vi "Main.vi"(7 "sweep rate, /min":dbl=0.2, 8 "sweep to:":dbl=-0.5, 9 "sweep":T6(radio)=enum."time_sweep") -> ()   [LabVIEW 2017] (continued)
                  n4093 = property on="data" class="Arr (strict)"() -> ("Value"=w5493:dbl[])  [unwired: 2 in, 2 out]
                  n4094 = case shown="True" w5491 {
                    tunnel: w5493 -> [w5494 w5497]
                    tunnel: [w5494 w5496] -> w5492
                    frame False {
                      # "We are not recording Step Value if it is linetrace"
                    }
                    frame True {
                      # "We are recording Step Value if it is mapping"
                      n4095 = property on="Current Hyper Value" class="DigNum (strict)"() -> ("Value"=w5495:dbl)  [unwired: 2 in, 2 out]
                      n4096 = Build Array (concatenate)(w5497, w5495) -> (w5496:dbl[])
                    }
                  }
                  n4097 = property on="data" class="Arr (strict)"("Value"=w5492) -> ()  [unwired: 2 in, 2 out]
                }
                frame #51 {
                  # "Record Step Value \nif it is mapping"
                  n4098 = property on="SuperHyper" class="Bool (strict)"() -> ("Value"=w5498:bool)  [unwired: 2 in, 2 out]
                  n4099 = property on="data" class="Arr (strict)"() -> ("Value"=w5500:dbl[])  [unwired: 2 in, 2 out]
                  n4100 = case shown="True" w5498 {
                    tunnel: w5500 -> [w5501 w5504]
                    tunnel: [w5501 w5503] -> w5499
                    frame False {
                      # "We are not recording Step Value if it is linetrace"
                    }
                    frame True {
                      # "We are recording SuperHyper_step if it is mapping"
                      n4101 = property on="Current SuperHyper Value" class="DigNum (strict)"() -> ("Value"=w5502:dbl)  [unwired: 2 in, 2 out]
                      n4102 = Build Array (concatenate)(w5504, w5502) -> (w5503:dbl[])
                    }
                  }
                  n4103 = property on="data" class="Arr (strict)"("Value"=w5499) -> ()  [unwired: 2 in, 2 out]
                }
              }
            }
            frame #4 {
              n4104 = property on="data" class="Arr (strict)"() -> ("Value"=w5505:dbl[])  [unwired: 2 in, 2 out]
            }
          }
          n4105 = stacked-sequence "add data to array" {
            tunnel: w4728 -> [w4740]
            tunnel: [w4739] -> w4727
            tunnel: w4726 -> [w4738]
            frame #0 {
              n4106 = Build Array (concatenate)(w4740, w4738) -> (w4739:dbl[][])
            }
          }
          n4107 = stacked-sequence "plot selected measurements" {
            seq-local: [_ w4763 _] -> [_ _ w4808]
            seq-local: [_ w4762 _] -> [_ _ w4809]
            tunnel: w4727 -> [_ w4761 _]
            frame #0 {
              n4108 = property on="XY Graph" class="XYGraph (strict)"("ActYScl"=0 ("Active Y Scale")) -> (error out=w4746:errorcluster)  [unwired: 2 in, 1 out]
              n4109 = property on="Show cursor" class="Bool (strict)"() -> ("Value"=w4741:bool)  [unwired: 2 in, 2 out]
              n4110 = property on="Xaxis" class="Ring (strict)"() -> ("Value"=w4751:u16)  [unwired: 2 in, 2 out]
              n4111 = property on="Yaxis" class="Ring (strict)"(error in=w4746) -> (error out=w4745:errorcluster, "RingText.Text"=w4744:string)  [unwired: 1 in, 1 out]
              n4112 = property on="XY Graph" class="XYGraph (strict)"("Cursor.Visible"=w4741) -> ()  [unwired: 2 in, 2 out]
              n4113 = property on="Figure_axis" class="Arr (strict)"() -> ("Value"=w4752:string[])  [unwired: 2 in, 2 out]
              n4114 = property on="XY Graph" class="XYGraph (strict)"(error in=w4745, "YScale.NameLbl.Text"=w4744) -> (error out=w4742:errorcluster)  [unwired: 1 in, 1 out]
              n4115 = property on="XY Graph" class="XYGraph (strict)"(error in=w4742, "ActYScl"=1 ("Active Y Scale")) -> (error out=w4748:errorcluster)  [unwired: 1 in, 1 out]
              n4116 = property on="Yright" class="Ring (strict)"(error in=w4748) -> (error out=w4749:errorcluster, "RingText.Text"=w4743:string)  [unwired: 1 in, 1 out]
              n4117 = Index Array(array=w4752, index=w4751) -> (element=w4753:string)
              n4118 = property on="XY Graph" class="XYGraph (strict)"("XScale.NameLbl.Text"=w4753) -> ()  [unwired: 2 in, 2 out]
              n4119 = property on="XY Graph" class="XYGraph (strict)"(error in=w4749, "YScale.NameLbl.Text"=w4743) -> ()  [unwired: 1 in, 2 out]
            }
            frame #1 {
              n4120 = local read "Xaxis"() -> (w4766:u16)
              n4121 = property on="Yright" class="Ring (strict)"() -> ("Value"=w4760:u16)  [unwired: 2 in, 2 out]
              n4122 = property on="Yright" class="Ring (strict)"() -> ("RingText.Text"=w4759:string)  [unwired: 2 in, 2 out]
              n4123 = property on="Xaxis" class="Ring (strict)"() -> ("RingText.Text"=w4765:string)  [unwired: 2 in, 2 out]
              n4124 = property on="Yaxis" class="Ring (strict)"() -> ("RingText.Text"=w4764:string)  [unwired: 2 in, 2 out]
              n4125 = local read "Yaxis"() -> (w4767:u16)
              n4126 = case shown="\"formula\"" w4759 {
                tunnel: [w4772 w4779] -> w4757
                tunnel: w4760 -> [_ w4778]
                tunnel: w4761 -> [w4773 w4777]
                tunnel: [w4771 errorcluster {"status"=FALSE, "code"=0, "source"=""} ("error out")] -> _
                frame "formula" {
                  n4127 = local read "formula_variables"() -> (w4774:string[])
                  n4128 = Transpose 2D Array(2D array=w4773) -> (transposed array=w4775:dbl[][])
                  n4129 = property on="Y_right_formula" class="Str"() -> ("Value"=w4770:string)  [unwired: 2 in, 2 out]
                  n4130 = call <vilib>:"Eval Multi-Variable Array.vi"("Variables"=w4774, "X Values"=w4775, "formula"=w4770) -> ("error out"=w4771:errorcluster, "Y Values"=w4772:dbl[])  [unwired: 1 in]
                }
                frame "0", Default {
                  n4131 = Index Array(array=w4777, index (col)=w4778) -> (element=w4779:dbl[])  [unwired: 1 in]
                }
              }
              n4132 = case shown="\"formula\"" w4765 {
                tunnel: [w4790 w4795] -> w4769
                tunnel: w4766 -> [w4793 _]
                tunnel: w4761 -> [w4792 w4799]
                tunnel: [errorcluster {"status"=FALSE, "code"=0, "source"=""} ("error out") w4796] -> w4763
                tunnel: [w4790 w4795] -> w4758
                frame "0", Default {
                  n4133 = Index Array(array=w4792, index (col)=w4793) -> (element=w4790:dbl[])  [unwired: 1 in]
                }
                frame "formula" {
                  n4134 = local read "formula_variables"() -> (w4798:string[])
                  n4135 = Transpose 2D Array(2D array=w4799) -> (transposed array=w4797:dbl[][])
                  n4136 = property on="X_axis_formula" class="Str"() -> ("Value"=w4794:string)  [unwired: 2 in, 2 out]
                  n4137 = call <vilib>:"Eval Multi-Variable Array.vi"("Variables"=w4798, "X Values"=w4797, "formula"=w4794) -> ("error out"=w4796:errorcluster, "Y Values"=w4795:dbl[])  [unwired: 1 in]
                }
              }
              n4138 = case shown="\"formula\"" w4764 {
                tunnel: [w4782 w4789] -> w4768
                tunnel: w4767 -> [_ w4788]
                tunnel: w4761 -> [w4783 w4787]
                tunnel: [w4781 errorcluster {"status"=FALSE, "code"=0, "source"=""} ("error out")] -> w4762
                frame "formula" {
                  n4139 = local read "formula_variables"() -> (w4784:string[])
                  n4140 = Transpose 2D Array(2D array=w4783) -> (transposed array=w4785:dbl[][])
                  n4141 = property on="Y_left_formula" class="Str"() -> ("Value"=w4780:string)  [unwired: 2 in, 2 out]
                  n4142 = call <vilib>:"Eval Multi-Variable Array.vi"("Variables"=w4784, "X Values"=w4785, "formula"=w4780) -> ("error out"=w4781:errorcluster, "Y Values"=w4782:dbl[])  [unwired: 1 in]
                }
                frame "0", Default {
                  n4143 = Index Array(array=w4787, index (col)=w4788) -> (element=w4789:dbl[])  [unwired: 1 in]
                }
              }
              n4144 = Bundle("Y Values"=w4769, "Y Values"=w4768) -> (w4756:cluster{"Y Values":dbl[], "Y Values":dbl[]})  [unwired: 1 in]
              n4145 = Bundle("Y Values"=w4758, "Y Values"=w4757) -> (w4755:cluster{"Y Values":dbl[], "Y Values":dbl[]})  [unwired: 1 in]
              n4146 = Build Array(w4756, w4755) -> (w4754:cluster{"Y Values":dbl[], "Y Values":dbl[]}[])
              n4147 = property on="XY Graph" class="XYGraph (strict)"("Value"=w4754) -> ()  [unwired: 2 in, 2 out]
            }
            frame #2 {
              # "show if formula \nis wrong"
              n4148 = property on="Yaxis" class="Ring (strict)"() -> ("RingText.Text"=w4805:string)  [unwired: 2 in, 2 out]
              n4149 = property on="XY Graph" class="XYGraph (strict)"("Active Plot"=u32 0, "Plot.Plot Name"=w4805) -> (error out=w4806:errorcluster)  [unwired: 2 in, 1 out]
              n4150 = property on="Yright" class="Ring (strict)"() -> ("RingText.Text"=w4803:string)  [unwired: 2 in, 2 out]
              n4151 = property on="XY Graph" class="XYGraph (strict)"(error in=w4806, "Active Plot"=u32 1, "Plot.Plot Name"=w4803) -> ()  [unwired: 1 in, 2 out]
              n4152 = Unbundle By Name(w4809) -> ("status"=w4802:bool)
              n4153 = Unbundle By Name(w4808) -> ("status"=w4801:bool)
              n4154 = Unbundle By Name(w4808) -> ("status"=w4800:bool)
              n4155 = property on="status 3" class="Bool (strict)"("Value"=w4800) -> ()  [unwired: 2 in, 2 out]
              n4156 = property on="status 2" class="Bool (strict)"("Value"=w4802) -> ()  [unwired: 2 in, 2 out]
              n4157 = property on="status" class="Bool (strict)"("Value"=w4801) -> ()  [unwired: 2 in, 2 out]
            }
          }
          n4158 = stacked-sequence "set next value in the sweep" {
            tunnel: w4737 -> [w5511 _]
            tunnel: [w5511 _] -> w4736
            tunnel: w4734 -> [_ w5629]
            tunnel: w4732 -> [w5514 _]
            frame #0 {
              n4159 = local read "sweep"() -> (w5517:T6)
              n4160 = property on="Sweep Channel" class="DigNum (strict)"("Value"=w5511) -> ()  [unwired: 2 in, 2 out]
              n4161 = property on="sweep value" class="DigNum (strict)"("Value"=w5511) -> ()  [unwired: 2 in, 2 out]
              n4162 = case shown="\"iPS\"" w5517 {
                tunnel: w5511 -> [w5530 w5538 w5544 w5553 w5575 _ w5577 w5600 w5623]
                tunnel: w5514 -> [_ _ _ w5552 _ _ _ _ _]
                frame "2400_1" {
                  # "sweep voltage on 2400 1"
                  n4163 = local read "2400 1 addr"() -> (w5532:u8)
                  n4164 = Number To Fractional String(number=w5530) -> (F-format string=w5536:string)  [unwired: 3 in]
                  n4165 = Concatenate Strings(":INIT:IMM; :SOUR:VOLT:LEV:IMM:AMPL " ("data"), w5536) -> (w5534:string)
                  n4166 = Number To Decimal String(number=w5532) -> (decimal integer string=w5531:string)  [unwired: 1 in]
                  n4167 = GPIB Write(0:w5531, 1:w5534, 2:i16 1 ("mode (0)")) -> ()  [unwired: 2 in, 2 out]
                }
                frame "2400_2" {
                  # "sweep curr on 2400 2"
                  n4168 = Number To Fractional String(number=w5538) -> (F-format string=w5543:string)  [unwired: 3 in]
                  n4169 = local read "2400 2 addr"() -> (w5540:u8)
                  n4170 = Concatenate Strings(":INIT:IMM; :SOUR:CURR:LEV:IMM:AMPL " ("data"), w5543) -> (w5541:string)
                  n4171 = Number To Decimal String(number=w5540) -> (decimal integer string=w5539:string)  [unwired: 1 in]
                  n4172 = GPIB Write(0:w5539, 1:w5541, 2:i16 1 ("mode (0)")) -> ()  [unwired: 2 in, 2 out]
                }
                frame "2400_3" {
                  # "sweep voltage on 2400 3"
                  n4173 = local read "2400 3 addr"() -> (w5546:u8)
                  n4174 = Number To Fractional String(number=w5544) -> (F-format string=w5550:string)  [unwired: 3 in]
                  n4175 = Concatenate Strings(":INIT:IMM; :SOUR:VOLT:LEV:IMM:AMPL " ("data"), w5550) -> (w5548:string)
                  n4176 = Number To Decimal String(number=w5546) -> (decimal integer string=w5545:string)  [unwired: 1 in]
                  n4177 = GPIB Write(0:w5545, 1:w5548, 2:i16 1 ("mode (0)")) -> ()  [unwired: 2 in, 2 out]
                }
                frame "2636a_smua" {
                  n4178 = property on="sweep 2" class="Bool (strict)"() -> ("Value"=w5551:bool)  [unwired: 2 in, 2 out]
                  n4179 = case shown="False" w5551 {
                    tunnel: w5553 -> [w5558 w5571]
                    tunnel: w5552 -> [w5555 _]
                    frame True {
                      w5556 = 30.0 ("y")
                      n4180 = Subtract(x=w5558, y=w5555) -> (x-y=w5557:dbl)
                      n4181 = Divide(x=w5557, y=w5556) -> (x/y=w5554:dbl)
                      n4182 = for {
                        N: w5556 -> [_]
                        tunnel: w5555 -> [w5564]
                        tunnel: w5554 -> [w5562]
                        i -> [w5563]
                        n4183 = Multiply(x=w5562, y=w5563) -> (x*y=w5561:dbl)
                        n4184 = local read "2336A addr"() -> (w5566:refnum<visa-resource-name>)
                        n4185 = Add(x=w5561, y=w5564) -> (x+y=w5560:dbl)
                        n4186 = call "setLevel.vi"("VISA resource name 2"=w5566, "Source"=Source."Voltage", "Channel"=Channel."a", "SourceLevel"=w5560) -> ()  [unwired: 1 in, 3 out]
                        n4187 = Wait (ms)(milliseconds to wait=u32 12) -> ()  [unwired: 1 out]
                      }
                    }
                    frame False {
                      # "sweep voltage on 2636a smua"
                      n4188 = local read "2336A addr"() -> (w5569:refnum<visa-resource-name>)
                      n4189 = call "setLevel.vi"("VISA resource name 2"=w5569, "Source"=Source."Voltage", "Channel"=Channel."a", "SourceLevel"=w5571) -> ()  [unwired: 1 in, 3 out]
                    }
                  }
                }
                frame "2636a_smub" {
                  # "sweep voltage on 2636b smua"
                  n4190 = local read "2336A addr"() -> (w5572:refnum<visa-resource-name>)
                  n4191 = call "setLevel.vi"("VISA resource name 2"=w5572, "Source"=Source."Voltage", "Channel"=Channel."b", "SourceLevel"=w5575) -> ()  [unwired: 1 in, 3 out]
                }
                frame "time_sweep", Default {
                  # "do not sweep, just time"
                }
                frame "iPS" {
                  n4192 = property on="Sweep B" class="Bool (strict)"() -> ("Value"=w5576:bool)  [unwired: 2 in, 2 out]
                  n4193 = case shown="False" w5576 {
                    tunnel: w5577 -> [_ w5578]
                    frame False {
                    }
                    frame True {
                      n4194 = stacked-sequence {
                        tunnel: w5578 -> [w5579 _ w5589 w5591]
                        frame #0 {
                          n4195 = local read "iPS_addr_sweep"() -> (w5581:refnum<visa-resource-name>)
                          n4196 = call "iPSset.vi"("Target Field, T"=w5579, "iPSSetCtrl"=iPSsetCtrl."Set Target Field", "VISA resource name"=w5581) -> ()  [unwired: 5 in, 4 out]
                        }
                        frame #1 {
                          n4197 = local read "iPS_addr_sweep"() -> (w5584:refnum<visa-resource-name>)
                          n4198 = call "iPSset.vi"("Field Rate, T/min"=0.15, "iPSSetCtrl"=iPSsetCtrl."Set Target Field Rate", "VISA resource name"=w5584) -> ()  [unwired: 5 in, 4 out]
                        }
                        frame #2 {
                          n4199 = Not Equal To 0?(x=w5589) -> (x != 0?=w5587:bool)
                          n4200 = local read "iPS_addr_sweep"() -> (w5590:refnum<visa-resource-name>)
                          n4201 = Select(t=iPSsetCtrl."Go to Field" ("iPSSetCtrl"), s=w5587, f=iPSsetCtrl."Go to Field" ("iPSSetCtrl")) -> (s? t:f=w5585:T18)
                          n4202 = call "iPSset.vi"("iPSSetCtrl"=w5585, "VISA resource name"=w5590) -> ()  [unwired: 6 in, 4 out]
                        }
                        frame #3 {
                          n4203 = while {
                            tunnel: w5591 -> [w5593]
                            stop <- w5597 stop-if-true
                            n4204 = property on="iPS _addr_step" class="VISAName"() -> ("Value"=w5596:refnum<visa-resource-name>)  [unwired: 2 in, 2 out]
                            n4205 = call "iPSread.vi"("iPSreadCtrl"=iPSreadCtrl."MagnetField", "VISA resource name"=w5596) -> ("number"=w5595:dbl)  [unwired: 6 in, 3 out]
                            n4206 = Subtract(x=w5595, y=w5593) -> (x-y=w5599:dbl)
                            n4207 = property on="Tolerance_Sweep" class="DigNum (strict)"() -> ("Value"=w5594:dbl)  [unwired: 2 in, 2 out]
                            n4208 = Absolute Value(x=w5599) -> (abs(x)=w5598:dbl)
                            n4209 = Less Or Equal?(x=w5598, y=w5594) -> (x <= y?=w5597:bool)
                          }
                        }
                      }
                    }
                  }
                }
                frame "iTC" {
                  n4210 = stacked-sequence {
                    tunnel: w5600 -> [w5601 w5608 w5614]
                    frame #0 {
                      n4211 = property on="iTC_addr_step" class="VISAName"() -> ("Value"=w5607:refnum<visa-resource-name>)  [unwired: 2 in, 2 out]
                      n4212 = Decrement(x=w5601) -> (x-1=w5603:dbl)
                      n4213 = Less Or Equal To 0?(x=w5603) -> (x <= 0?=w5605:bool)
                      n4214 = Select(t=0.0, s=w5605, f=w5603) -> (s? t:f=w5602:dbl)
                      n4215 = call "iTCset.vi"("Set Point"=w5602, "iTCSetCtrl"=iTCsetCtrl."Set VTI Temp", "VISA resource name"=w5607) -> ()  [unwired: 5 in, 4 out]
                    }
                    frame #1 {
                      n4216 = property on="iTC_addr_step" class="VISAName"() -> ("Value"=w5613:refnum<visa-resource-name>)  [unwired: 2 in, 2 out]
                      n4217 = Less Or Equal To 0?(x=w5608) -> (x <= 0?=w5611:bool)
                      n4218 = Select(t=0.0, s=w5611, f=w5608) -> (s? t:f=w5609:dbl)
                      n4219 = call "iTCset.vi"("Set Point"=w5609, "iTCSetCtrl"=iTCsetCtrl."Set Sample Temp", "VISA resource name"=w5613) -> ()  [unwired: 5 in, 4 out]
                    }
                    frame #2 {
                      n4220 = while {
                        tunnel: w5614 -> [w5616]
                        stop <- w5617 stop-if-true
                        n4221 = property on="iTC_addr_step" class="VISAName"() -> ("Value"=w5622:refnum<visa-resource-name>)  [unwired: 2 in, 2 out]
                        n4222 = call "iTCread.vi"("VISA resource name"=w5622, "iTCreadCtrl"=iTCreadCtrl."Sample Temp") -> ("number"=w5620:dbl)  [unwired: 5 in, 3 out]
                        n4223 = Subtract(x=w5620, y=w5616) -> (x-y=w5619:dbl)
                        n4224 = property on="Tolerance_Sweep" class="DigNum (strict)"() -> ("Value"=w5615:dbl)  [unwired: 2 in, 2 out]
                        n4225 = Absolute Value(x=w5619) -> (abs(x)=w5618:dbl)
                        n4226 = Less?(x=w5618, y=w5615) -> (x < y?=w5617:bool)
                      }
                    }
                  }
                }
                frame "2461" {
                  w5624 = u16 1 items=["Volts", "Current"] ("Function (0: Volts)")
                  n4227 = property on="2461_addr_sweep" class="VISAName"() -> ("Value"=w5625:refnum<visa-resource-name>)  [unwired: 2 in, 2 out]
                  n4228 = call <instrlib>:"Configure Source Level.vi"("Source Level (1.0)"=w5623, "Function (0: Volts)"=w5624, "VISA resource name"=w5625) -> ()  [unwired: 7 in, 2 out]
                }
              }
              n4229 = property on="Offset" class="DigNum (strict)"() -> ("Value"=w5513:dbl)  [unwired: 2 in, 2 out]
              n4230 = property on="Slope" class="DigNum (strict)"() -> ("Value"=w5512:dbl)  [unwired: 2 in, 2 out]
              n4231 = Multiply(x=w5512, y=w5511) -> (x*y=w5515:dbl)
              n4232 = local read "sweep"() -> (w5510:T6)
              n4233 = property on="Lead Chanl" class="Enum (strict)"() -> ("Value"=w5509:T1)  [unwired: 2 in, 2 out]
              n4234 = property on="Double Sweep" class="Bool (strict)"() -> ("Value"=w5507:bool)  [unwired: 2 in, 2 out]
              n4235 = Add(x=w5513, y=w5515) -> (x+y=w5516:dbl)
              n4236 = Equal?(x=w5510, y=w5509) -> (x = y?=w5508:bool)
              n4237 = And(x=w5507, y=w5508) -> (x .and. y?=w5506:bool)
              n4238 = case shown="True" w5506 {
                tunnel: w5516 -> [_ w5518]
                frame False {
                }
                frame True {
                  n4239 = disable-structure shown="Enabled" {
                    disable-tunnel: w5518 -> [w5519 w5527]
                    frame Disabled {
                      # "sweep voltage on 2400 2"
                      n4240 = local read "2400 2 addr"() -> (w5520:u8)
                      n4241 = Number To Fractional String(number=w5519) -> (F-format string=w5521:string)  [unwired: 3 in]
                      n4242 = Concatenate Strings(":INIT:IMM; :SOUR:VOLT:LEV:IMM:AMPL " ("data"), w5521) -> (w5523:string)
                      n4243 = Number To Decimal String(number=w5520) -> (decimal integer string=w5524:string)  [unwired: 1 in]
                      n4244 = GPIB Write(0:w5524, 1:w5523, 2:i16 1 ("mode (0)")) -> ()  [unwired: 2 in, 2 out]
                    }
                    frame Enabled {
                      n4245 = property on="Slave Channel" class="Enum (strict)"() -> ("Value"=w5526:T2)  [unwired: 2 in, 2 out]
                      n4246 = local read "2336A addr"() -> (w5529:refnum<visa-resource-name>)
                      n4247 = call "setLevel.vi"("VISA resource name 2"=w5529, "Source"=Source."Voltage", "Channel"=w5526, "SourceLevel"=w5527) -> ()  [unwired: 1 in, 3 out]
                    }
                  }
                }
              }
            }
            frame #1 {
              # "calculate deliberate time delay for the next step"
              n4248 = Tick Count (ms)() -> (millisecond timer value=w5631:u32)
              n4249 = Subtract(x=w5631, y=w5629) -> (x-y=w5630:u32)
              n4250 = property on="time/point, sec" class="DigNum (strict)"() -> ("Value"=w5626:dbl)  [unwired: 2 in, 2 out]
              n4251 = Multiply(x=w5626, y=1000.0) -> (x*y=w5628:dbl)
              n4252 = Subtract(x=w5628, y=w5630) -> (x-y=w5627:dbl)
              n4253 = property on="time delay, ms" class="DigNum (strict)"("Value"=w5627) -> ()  [unwired: 2 in, 2 out]
            }
          }
          n4254 = Or(x=w4730, y="Stop Ramp") -> (x .or. y?=w4731:bool)
        }
        n4255 = stacked-sequence {
          tunnel: w3756 -> [_ _]
          tunnel: w3755 -> [_ w4716]
          frame #0 {
            n4256 = stacked-sequence {
              frame #0 {
                n4257 = local read "sweep"() -> (w4706:T6)
                n4258 = Equal?(x=w4706, y=T19."Radio Selection 7" ("sweep")) -> (x = y?=w4705:bool)
                n4259 = case shown="True" w4705 {
                  frame False {
                  }
                  frame True {
                    n4260 = local read "iPS_addr_sweep"() -> (w4707:refnum<visa-resource-name>)
                    n4261 = call "iPSset.vi"("iPSSetCtrl"=iPSsetCtrl."Hold", "VISA resource name"=w4707) -> ()  [unwired: 6 in, 4 out]
                  }
                }
              }
              frame #1 {
                n4262 = local read "2636A smua meas v"() -> (w4714:bool)
                n4263 = local read "2636A smub meas v"() -> (w4712:bool)
                n4264 = local read "2636A smub meas i"() -> (w4711:bool)
                n4265 = local read "2636A smua meas i"() -> (w4713:bool)
                n4266 = Compound Arithmetic op=OR(w4714, w4713, w4712, w4711) -> (w4710:bool)
                n4267 = property on="Stop Ramp" class="Bool"("DisabledEnum"=T12."Disabled and Grayed Out" ("Disabled")) -> ()  [unwired: 2 in, 2 out]
                n4268 = case shown="False" w4710 {
                  frame False {
                  }
                  frame True {
                    # "close session on 2636A"
                    n4269 = local read "2336A addr"() -> (w4715:refnum<visa-resource-name>)
                    n4270 = VISA Close(VISA resource name=w4715) -> ()  [unwired: 1 in, 1 out]
                  }
                }
              }
            }
          }
          frame #1 {
            n4271 = property on="Step Loop" class="Bool (strict)"() -> ("Value"=w4717:bool)  [unwired: 2 in, 2 out]
            n4272 = case shown="True" w4717 {
              tunnel: w4716 -> [w4721 w4722]
              frame False {
                w4719 = T12."Enabled" ("Disabled")
                n4273 = Enqueue Element(queue=w4721, element="Idle") -> ()  [unwired: 2 in, 3 out]
                n4274 = property on="sweep" class="RadioBtnsControl (strict)"("DisabledEnum"=w4719) -> ()  [unwired: 2 in, 2 out]
                n4275 = property on="2182A 1 addr" class="DigNum (strict)"("DisabledEnum"=w4719) -> ()  [unwired: 2 in, 2 out]
                n4276 = property on="2182A 2 addr" class="DigNum (strict)"("DisabledEnum"=w4719) -> ()  [unwired: 2 in, 2 out]
                n4277 = property on="2182A 3 addr" class="DigNum (strict)"("DisabledEnum"=w4719) -> ()  [unwired: 2 in, 2 out]
                n4278 = property on="2182A 4 addr" class="DigNum (strict)"("DisabledEnum"=w4719) -> ()  [unwired: 2 in, 2 out]
                n4279 = property on="2400 1 addr" class="DigNum (strict)"("DisabledEnum"=w4719) -> ()  [unwired: 2 in, 2 out]
                n4280 = property on="Sweep Down" class="Bool"("DisabledEnum"=w4719) -> ()  [unwired: 2 in, 2 out]
                n4281 = property on="2400 2 addr" class="DigNum (strict)"("DisabledEnum"=w4719) -> ()  [unwired: 2 in, 2 out]
                n4282 = property on="2400 3 addr" class="DigNum (strict)"("DisabledEnum"=w4719) -> ()  [unwired: 2 in, 2 out]
                n4283 = property on="2336A addr" class="VISAName"("DisabledEnum"=w4719) -> ()  [unwired: 2 in, 2 out]
                n4284 = property on="SR830 1 addr" class="DigNum (strict)"("DisabledEnum"=w4719) -> ()  [unwired: 2 in, 2 out]
                n4285 = property on="SR830 2 addr" class="DigNum (strict)"("DisabledEnum"=w4719) -> ()  [unwired: 2 in, 2 out]
                n4286 = property on="SR830 3 addr" class="DigNum (strict)"("DisabledEnum"=w4719) -> ()  [unwired: 2 in, 2 out]
                n4287 = property on="SR830 4 addr" class="DigNum (strict)"("DisabledEnum"=w4719) -> ()  [unwired: 2 in, 2 out]
                n4288 = property on="Stop Ramp" class="Bool"("DisabledEnum"=T12."Disabled and Grayed Out" ("Disabled")) -> ()  [unwired: 2 in, 2 out]
              }
              frame True {
                n4289 = stacked-sequence {
                  tunnel: w4722 -> [_ w4725]
                  frame #0 {
                    n4290 = property on="Sweep Direction" class="Str"("Value"="Sweep Down" ("Sweep Direction")) -> ()  [unwired: 2 in, 2 out]
                  }
                  frame #1 {
                    n4291 = Enqueue Element(queue=w4725, element="Step to Next Value") -> ()  [unwired: 2 in, 3 out]
                  }
                }
              }
            }
          }
        }
      }
      frame "Step to Next Value" {
        n4292 = property on="Table Index" class="DigNum (strict)"() -> ("Value"=w5647:dbl)  [unwired: 2 in, 2 out]
        n4293 = property on="Step values" class="Tbl (strict)"() -> ("Value"=w5646:string[][])  [unwired: 2 in, 2 out]
        n4294 = Equal?(x=w5647, y=0) -> (x = y?=w5643:bool)
        n4295 = case shown="True" w5643 {
          tunnel: w5647 -> [w5648 w5672]
          tunnel: cluster{"Row":i32, "Column":i32} {"Row"=0, "Column"=0} ("Active Cell:Active Cell") -> [w5652 w5675]
          frame False {
            w5655 = 0 ("Column")
            n4296 = property on="Change Sweep Range" class="Bool (strict)"() -> ("Value"=w5649:bool)  [unwired: 2 in, 2 out]
            n4297 = Decrement(x=w5648) -> (x-1=w5656:dbl)
            n4298 = Bundle By Name(cluster=w5652, "Row"=w5648, "Column"=w5655) -> (w5651:cluster{"Row":i32, "Column":i32})
            n4299 = case shown="True" w5649 {
              tunnel: w5648 -> [_ w5658]
              frame False {
              }
              frame True {
                w5659 = 1 ("Column")
                w5671 = 0 ("Column")
                n4300 = Decrement(x=w5658) -> (x-1=w5670:dbl)
                n4301 = Bundle By Name(cluster=cluster{"Row":i32, "Column":i32} {"Row"=0, "Column"=0} ("Active Cell:Active Cell"), "Row"=w5658, "Column"=w5671) -> (w5668:cluster{"Row":i32, "Column":i32})
                n4302 = Decrement(x=w5658) -> (x-1=w5660:dbl)
                n4303 = Bundle By Name(cluster=w5668, "Row"=w5670, "Column"=w5671) -> (w5667:cluster{"Row":i32, "Column":i32})
                n4304 = Bundle By Name(cluster=cluster{"Row":i32, "Column":i32} {"Row"=0, "Column"=0} ("Active Cell:Active Cell"), "Row"=w5658, "Column"=w5659) -> (w5661:cluster{"Row":i32, "Column":i32})
                n4305 = Bundle By Name(cluster=w5661, "Row"=w5660, "Column"=w5659) -> (w5662:cluster{"Row":i32, "Column":i32})
                n4306 = property on="Down          Up" class="Tbl (strict)"("Active Cell"=w5667, "Cell BG Color"=u32 16711680 ("Active Cell:Cell Background Color")) -> ()  [unwired: 2 in, 2 out]
                n4307 = property on="Down          Up" class="Tbl (strict)"("Active Cell"=w5668, "Cell BG Color"=u32 16776072 ("Active Cell:Cell Background Color")) -> ()  [unwired: 2 in, 2 out]
                n4308 = property on="Down          Up" class="Tbl (strict)"("Active Cell"=w5662, "Cell BG Color"=u32 16711680 ("Active Cell:Cell Background Color")) -> ()  [unwired: 2 in, 2 out]
                n4309 = property on="Down          Up" class="Tbl (strict)"("Active Cell"=w5661, "Cell BG Color"=u32 16776072 ("Active Cell:Cell Background Color")) -> ()  [unwired: 2 in, 2 out]
              }
            }
            n4310 = Bundle By Name(cluster=w5651, "Row"=w5656, "Column"=w5655) -> (w5650:cluster{"Row":i32, "Column":i32})
            n4311 = property on="Step values" class="Tbl (strict)"("Active Cell"=w5651, "Cell BG Color"=u32 16776072 ("Active Cell:Cell Background Color")) -> ()  [unwired: 2 in, 2 out]
            n4312 = property on="Step values" class="Tbl (strict)"("Active Cell"=w5650, "Cell BG Color"=u32 16711680 ("Active Cell:Cell Background Color")) -> ()  [unwired: 2 in, 2 out]
          }
          frame True {
            n4313 = property on="Change Sweep Range" class="Bool (strict)"() -> ("Value"=w5673:bool)  [unwired: 2 in, 2 out]
            n4314 = Bundle By Name(cluster=w5675, "Row"=w5672, "Column"=0) -> (w5674:cluster{"Row":i32, "Column":i32})
            n4315 = case shown="True" w5673 {
              tunnel: w5672 -> [_ w5683]
              frame False {
              }
              frame True {
                w5682 = cluster{"Row":i32, "Column":i32} {"Row"=0, "Column"=0} ("Active Cell:Active Cell")
                n4316 = Bundle By Name(cluster=w5682, "Row"=w5683, "Column"=1) -> (w5679:cluster{"Row":i32, "Column":i32})
                n4317 = Bundle By Name(cluster=w5682, "Row"=w5683, "Column"=0) -> (w5681:cluster{"Row":i32, "Column":i32})
                n4318 = property on="Down          Up" class="Tbl (strict)"("Active Cell"=w5681, "Cell BG Color"=u32 16776072 ("Active Cell:Cell Background Color")) -> ()  [unwired: 2 in, 2 out]
                n4319 = property on="Down          Up" class="Tbl (strict)"("Active Cell"=w5679, "Cell BG Color"=u32 16776072 ("Active Cell:Cell Background Color")) -> ()  [unwired: 2 in, 2 out]
              }
            }
            n4320 = property on="Step values" class="Tbl (strict)"("Active Cell"=w5674, "Cell BG Color"=u32 16776072 ("Active Cell:Cell Background Color")) -> ()  [unwired: 2 in, 2 out]
          }
        }
        n4321 = call <vilib>:"Space Constant.vi"() -> ("String"=w5641:string)
        n4322 = Index Array(array=w5646, index (row)=w5647, index (col)=0 ("disabled index (col)")) -> (element=w5640:string)
        n4323 = call <vilib>:"Search and Replace Pattern.vi"("string"=w5640, "regular expression (\"\")"=w5641, "replace string (\"\")"="" ("replace string (\"\")"), "replace all? (F)"=TRUE) -> ("result string"=w5644:string)  [unwired: 1 in, 1 out]
        n4324 = Equal?(x="", y=w5644) -> (x = y?=w5642:bool)
        n4325 = Fract/Exp String To Number(string=w5644) -> (number=w5645:dbl)  [unwired: 3 in, 1 out]
        n4326 = case shown="False" w5642 {
          tunnel: w5645 -> [w5686 _]
          tunnel: w5634 -> [w5687 w5917]
          frame False {
            # "When step values are not finished"
            n4327 = property on="Current Step Value" class="DigNum (strict)"("Value"=w5686) -> ()  [unwired: 2 in, 2 out]
            n4328 = stacked-sequence {
              tunnel: w5686 -> [w5688 _ _ _]
              tunnel: w5687 -> [_ _ _ w5914]
              frame #0 {
                # "1 = 2400 1\n2 = 2400 2\n\n4 = 2636a smua\n5 = 2636a smub\n6 = do not sweep, just time\n7 = iPS, magnetic field \n8 = iTC, temperature"
                # "set next value in the sweep"
                n4329 = property on="step" class="RadioBtnsControl (strict)"() -> ("Value"=w5689:T8)  [unwired: 2 in, 2 out]
                n4330 = case shown="\"2461_Curr\"" w5689 {
                  tunnel: w5688 -> [w5691 w5698 w5704 w5734 w5764 w5767 w5835 w5879]
                  frame "V2400_1_Step" {
                    # "sweep voltage on 2400 1"
                    n4331 = property on="2400_1_addr_step" class="DigNum (strict)"() -> ("Value"=w5690:u8)  [unwired: 2 in, 2 out]
                    n4332 = Number To Fractional String(number=w5691) -> (F-format string=w5696:string)  [unwired: 3 in]
                    n4333 = Concatenate Strings(":INIT:IMM; :SOUR:VOLT:LEV:IMM:AMPL " ("data"), w5696) -> (w5694:string)
                    n4334 = Number To Decimal String(number=w5690) -> (decimal integer string=w5692:string)  [unwired: 1 in]
                    n4335 = GPIB Write(0:w5692, 1:w5694, 2:i16 1 ("mode (0)")) -> ()  [unwired: 2 in, 2 out]
                  }
                  frame "V2400_2_step" {
                    # "sweep voltage on 2400 2"
                    n4336 = property on="2400_2_addr_step" class="DigNum (strict)"() -> ("Value"=w5697:u8)  [unwired: 2 in, 2 out]
                    n4337 = Number To Fractional String(number=w5698) -> (F-format string=w5703:string)  [unwired: 3 in]
                    n4338 = Concatenate Strings(":INIT:IMM; :SOUR:CURR:LEV:IMM:AMPL " ("data"), w5703) -> (w5701:string)
                    n4339 = Number To Decimal String(number=w5697) -> (decimal integer string=w5699:string)  [unwired: 1 in]
                    n4340 = GPIB Write(0:w5699, 1:w5701, 2:i16 1 ("mode (0)")) -> ()  [unwired: 2 in, 2 out]
                  }
                  frame "2636_smua_step" {
                    # "sweep voltage on 2636a smua"
                    n4341 = property on="Step Channel" class="DigNum (strict)"() -> ("Value"=w5707:dbl)  [unwired: 2 in, 2 out]
                    n4342 = property on="Mini steps" class="DigNum (strict)"() -> ("Value"=w5705:dbl)  [unwired: 2 in, 2 out]
                    n4343 = property on="2336A_addr_step" class="VISAName"() -> ("Value"=w5706:refnum<visa-resource-name>)  [unwired: 2 in, 2 out]
                    n4344 = Subtract(x=w5704, y=w5707) -> (x-y=w5708:dbl)
                    n4345 = Divide(x=w5708, y=w5705) -> (x/y=w5709:dbl)
                    n4346 = for {
                      N: w5705 -> [_]
                      tunnel: w5707 -> [w5723]
                      tunnel: w5709 -> [w5722]
                      tunnel: w5706 -> [w5719]
                      i -> [w5718]
                      n4347 = Increment(x=w5718) -> (x+1=w5717:i32)
                      n4348 = Multiply(x=w5722, y=w5717) -> (x*y=w5721:dbl)
                      n4349 = Add(x=w5721, y=w5723) -> (x+y=w5715:dbl)
                      n4350 = property on="Lead Chanl_step" class="Enum (strict)"() -> ("Value"=w5714:T7)  [unwired: 2 in, 2 out]
                      n4351 = property on="step" class="RadioBtnsControl (strict)"() -> ("Value"=w5713:T8)  [unwired: 2 in, 2 out]
                      n4352 = call "setLevel.vi"("VISA resource name 2"=w5719, "Source"=Source."Voltage", "Channel"=Channel."a", "SourceLevel"=w5715) -> ("VISA resource name"=w5716:refnum<visa-resource-name>)  [unwired: 1 in, 2 out]
                      n4353 = property on="diagonal step" class="Bool (strict)"() -> ("Value"=w5712:bool)  [unwired: 2 in, 2 out]
                      n4354 = Wait (ms)(milliseconds to wait=u32 12) -> ()  [unwired: 1 out]
                      n4355 = Equal?(x=w5714, y=w5713) -> (x = y?=w5711:bool)
                      n4356 = property on="Current Step Value" class="DigNum (strict)"("Value"=w5715) -> ()  [unwired: 2 in, 2 out]
                      n4357 = And(x=w5712, y=w5711) -> (x .and. y?=w5710:bool)
                      n4358 = case shown="True" w5710 {
                        tunnel: w5715 -> [_ w5733]
                        tunnel: w5716 -> [_ w5728]
                        frame False {
                        }
                        frame True {
                          n4359 = property on="Step Slope" class="DigNum (strict)"() -> ("Value"=w5727:dbl)  [unwired: 2 in, 2 out]
                          n4360 = property on="Step Offset" class="DigNum (strict)"() -> ("Value"=w5726:dbl)  [unwired: 2 in, 2 out]
                          n4361 = Multiply(x=w5733, y=w5727) -> (x*y=w5732:dbl)
                          n4362 = Add(x=w5732, y=w5726) -> (x+y=w5729:dbl)
                          n4363 = call "setLevel.vi"("VISA resource name 2"=w5728, "Source"=Source."Voltage", "Channel"=Channel."b", "SourceLevel"=w5729) -> ()  [unwired: 1 in, 3 out]
                        }
                      }
                    }
                  }
                  frame "2636_smub_step" {
                    # "sweep voltage on 2636a smua"
                    n4364 = property on="Step Channel" class="DigNum (strict)"() -> ("Value"=w5737:dbl)  [unwired: 2 in, 2 out]
                    n4365 = property on="Mini steps" class="DigNum (strict)"() -> ("Value"=w5735:dbl)  [unwired: 2 in, 2 out]
                    n4366 = property on="2336A_addr_step" class="VISAName"() -> ("Value"=w5736:refnum<visa-resource-name>)  [unwired: 2 in, 2 out]
                    n4367 = Subtract(x=w5734, y=w5737) -> (x-y=w5738:dbl)
                    n4368 = Divide(x=w5738, y=w5735) -> (x/y=w5739:dbl)
                    n4369 = for {
                      N: w5735 -> [_]
                      tunnel: w5737 -> [w5753]
                      tunnel: w5739 -> [w5752]
                      tunnel: w5736 -> [w5749]
                      i -> [w5748]
                      n4370 = Increment(x=w5748) -> (x+1=w5747:i32)
                      n4371 = Multiply(x=w5752, y=w5747) -> (x*y=w5751:dbl)
                      n4372 = Add(x=w5751, y=w5753) -> (x+y=w5745:dbl)
                      n4373 = property on="Lead Chanl_step" class="Enum (strict)"() -> ("Value"=w5744:T7)  [unwired: 2 in, 2 out]
                      n4374 = property on="step" class="RadioBtnsControl (strict)"() -> ("Value"=w5743:T8)  [unwired: 2 in, 2 out]
                      n4375 = call "setLevel.vi"("VISA resource name 2"=w5749, "Source"=Source."Voltage", "Channel"=Channel."b", "SourceLevel"=w5745) -> ("VISA resource name"=w5746:refnum<visa-resource-name>)  [unwired: 1 in, 2 out]
                      n4376 = property on="diagonal step" class="Bool (strict)"() -> ("Value"=w5742:bool)  [unwired: 2 in, 2 out]
                      n4377 = Wait (ms)(milliseconds to wait=u32 12) -> ()  [unwired: 1 out]
                      n4378 = Equal?(x=w5744, y=w5743) -> (x = y?=w5741:bool)
                      n4379 = And(x=w5742, y=w5741) -> (x .and. y?=w5740:bool)
                      n4380 = property on="Current Step Value" class="DigNum (strict)"("Value"=w5745) -> ()  [unwired: 2 in, 2 out]
                      n4381 = case shown="True" w5740 {
                        tunnel: w5745 -> [_ w5763]
                        tunnel: w5746 -> [_ w5758]
                        frame False {
                        }
                        frame True {
                          n4382 = property on="Step Slope" class="DigNum (strict)"() -> ("Value"=w5757:dbl)  [unwired: 2 in, 2 out]
                          n4383 = property on="Step Offset" class="DigNum (strict)"() -> ("Value"=w5756:dbl)  [unwired: 2 in, 2 out]
                          n4384 = Multiply(x=w5763, y=w5757) -> (x*y=w5762:dbl)
                          n4385 = Add(x=w5762, y=w5756) -> (x+y=w5759:dbl)
                          n4386 = call "setLevel.vi"("VISA resource name 2"=w5758, "Source"=Source."Voltage", "Channel"=Channel."a", "SourceLevel"=w5759) -> ()  [unwired: 1 in, 3 out]
                        }
                      }
                    }
                  }
                  frame "time_step", Default {
                    # "do not sweep, just time"
                    n4387 = case shown="True" "Change Doule Sweep OffSet" {
                      tunnel: w5764 -> [_ w5766]
                      frame False {
                      }
                      frame True {
                        n4388 = property on="Offset" class="DigNum (strict)"("Value"=w5766) -> ()  [unwired: 2 in, 2 out]
                      }
                    }
                  }
                  frame "iPS_step" {
                    # "step magnetic field"
                    n4389 = stacked-sequence {
                      tunnel: w5767 -> [_ _ _ _ w5780 _ _ _ w5793 _ w5801 _]
                      frame #0 {
                        n4390 = property on="Table Index" class="DigNum (strict)"() -> ("Value"=w5770:dbl)  [unwired: 2 in, 2 out]
                        n4391 = Equal?(x=w5770, y=0.0) -> (x = y?=w5768:bool)
                        n4392 = case shown="True" w5768 {
                          frame False {
                          }
                          frame True {
                            n4393 = property on="iPS _addr_step" class="VISAName"() -> ("Value"=w5774:refnum<visa-resource-name>)  [unwired: 2 in, 2 out]
                            n4394 = property on="FieldRate(T/min)" class="DigNum (strict)"() -> ("Value"=w5771:dbl)  [unwired: 2 in, 2 out]
                            n4395 = call "iPSset.vi"("Field Rate, T/min"=w5771, "iPSSetCtrl"=iPSsetCtrl."Set Target Field Rate", "VISA resource name"=w5774) -> ("VISA resource name out"=w5772:refnum<visa-resource-name>)  [unwired: 5 in, 3 out]
                            n4396 = property on="iPS _addr_step" class="VISAName"("Value"=w5772) -> ()  [unwired: 2 in, 2 out]
                          }
                        }
                      }
                      frame #1 {
                        n4397 = Wait (ms)(milliseconds to wait=u32 500) -> ()  [unwired: 1 out]
                      }
                      frame #2 {
                        n4398 = property on="iPS _addr_step" class="VISAName"() -> ("Value"=w5778:refnum<visa-resource-name>)  [unwired: 2 in, 2 out]
                        n4399 = call "iPSset.vi"("iPSSetCtrl"=iPSsetCtrl."Hold", "VISA resource name"=w5778) -> ("VISA resource name out"=w5776:refnum<visa-resource-name>)  [unwired: 6 in, 3 out]
                        n4400 = property on="iPS _addr_step" class="VISAName"("Value"=w5776) -> ()  [unwired: 2 in, 2 out]
                      }
                      frame #3 {
                        n4401 = Wait (ms)(milliseconds to wait=u32 500) -> ()  [unwired: 1 out]
                      }
                      frame #4 {
                        n4402 = property on="iPS _addr_step" class="VISAName"() -> ("Value"=w5783:refnum<visa-resource-name>)  [unwired: 2 in, 2 out]
                        n4403 = call "iPSset.vi"("Target Field, T"=w5780, "iPSSetCtrl"=iPSsetCtrl."Set Target Field", "VISA resource name"=w5783) -> ("VISA resource name out"=w5781:refnum<visa-resource-name>)  [unwired: 5 in, 3 out]
                        n4404 = property on="iPS _addr_step" class="VISAName"("Value"=w5781) -> ()  [unwired: 2 in, 2 out]
                      }
                      frame #5 {
                        n4405 = Wait (ms)(milliseconds to wait=u32 500) -> ()  [unwired: 1 out]
                      }
                      frame #6 {
                        n4406 = property on="iPS _addr_step" class="VISAName"() -> ("Value"=w5787:refnum<visa-resource-name>)  [unwired: 2 in, 2 out]
                        n4407 = call "iPSset.vi"("iPSSetCtrl"=iPSsetCtrl."Hold", "VISA resource name"=w5787) -> ("VISA resource name out"=w5785:refnum<visa-resource-name>)  [unwired: 6 in, 3 out]
                        n4408 = property on="iPS _addr_step" class="VISAName"("Value"=w5785) -> ()  [unwired: 2 in, 2 out]
                      }
                      frame #7 {
                        n4409 = Wait (ms)(milliseconds to wait=u32 500) -> ()  [unwired: 1 out]
                      }
                      frame #8 {
                        n4410 = Equal To 0?(x=w5793) -> (x = 0?=w5792:bool)
                        n4411 = property on="iPS _addr_step" class="VISAName"() -> ("Value"=w5794:refnum<visa-resource-name>)  [unwired: 2 in, 2 out]
                        n4412 = Select(t=iPSsetCtrl."Go to Zero" ("iPSSetCtrl"), s=w5792, f=iPSsetCtrl."Go to Field" ("iPSSetCtrl")) -> (s? t:f=w5789:T18)
                        n4413 = call "iPSset.vi"("iPSSetCtrl"=w5789, "VISA resource name"=w5794) -> ()  [unwired: 6 in, 4 out]
                      }
                      frame #9 {
                        n4414 = Wait (ms)(milliseconds to wait=u32 500) -> ()  [unwired: 1 out]
                      }
                      frame #10 {
                        n4415 = while {
                          tunnel: w5801 -> [w5832]
                          stop <- w5824 stop-if-true
                          n4416 = property on="iPS _addr_step" class="VISAName"() -> ("Value"=w5829:refnum<visa-resource-name>)  [unwired: 2 in, 2 out]
                          n4417 = call "iPSread.vi"("iPSreadCtrl"=iPSreadCtrl."MagnetField", "VISA resource name"=w5829) -> ("number"=w5825:dbl, "VISA resource name out"=w5827:refnum<visa-resource-name>)  [unwired: 6 in, 2 out]
                          n4418 = property on="iPS _addr_step" class="VISAName"("Value"=w5827) -> ()  [unwired: 2 in, 2 out]
                          n4419 = property on="Tolerance_Step" class="DigNum (strict)"() -> ("Value"=w5826:dbl)  [unwired: 2 in, 2 out]
                          n4420 = Wait (ms)(milliseconds to wait=u32 500) -> ()  [unwired: 1 out]
                          n4421 = Subtract(x=w5825, y=w5832) -> (x-y=w5831:dbl)
                          n4422 = Absolute Value(x=w5831) -> (abs(x)=w5830:dbl)
                          n4423 = Less Or Equal?(x=w5830, y=w5826) -> (x <= y?=w5824:bool)
                          n4424 = property on="Step Channel" class="DigNum (strict)"("Value"=w5825) -> ()  [unwired: 2 in, 2 out]
                          n4425 = property on="at field" class="Bool (strict)"("Value"=w5824) -> ()  [unwired: 2 in, 2 out]
                        }
                        n4426 = property on="Lead Chanl_step" class="Enum (strict)"() -> ("Value"=w5800:T7)  [unwired: 2 in, 2 out]
                        n4427 = property on="step" class="RadioBtnsControl (strict)"() -> ("Value"=w5799:T8)  [unwired: 2 in, 2 out]
                        n4428 = property on="diagonal step" class="Bool (strict)"() -> ("Value"=w5798:bool)  [unwired: 2 in, 2 out]
                        n4429 = Equal?(x=w5800, y=w5799) -> (x = y?=w5797:bool)
                        n4430 = And(x=w5798, y=w5797) -> (x .and. y?=w5796:bool)
                        n4431 = case shown="True" w5796 {
                          tunnel: w5801 -> [_ w5806]
                          frame False {
                          }
                          frame True {
                            n4432 = property on="Channel" class="Enum (strict)"() -> ("Value"=w5804:T2)  [unwired: 2 in, 2 out]
                            n4433 = property on="2336A_addr_step" class="VISAName"() -> ("Value"=w5805:refnum<visa-resource-name>)  [unwired: 2 in, 2 out]
                            n4434 = property on="Step Offset" class="DigNum (strict)"() -> ("Value"=w5811:dbl)  [unwired: 2 in, 2 out]
                            n4435 = property on="Step Slope" class="DigNum (strict)"() -> ("Value"=w5812:dbl)  [unwired: 2 in, 2 out]
                            n4436 = call "SinglePointMeasurement.vi"("Measure"=Measure."Voltage", "Channel"=w5804, "VISA resource name 2"=w5805) -> ("Measuremet"=w5802:dbl)  [unwired: 3 in, 4 out]
                            n4437 = Multiply(x=w5806, y=w5812) -> (x*y=w5813:dbl)
                            n4438 = Add(x=w5813, y=w5811) -> (x+y=w5807:dbl)
                            n4439 = Subtract(x=w5807, y=w5802) -> (x-y=w5809:dbl)
                            n4440 = property on="Mini steps" class="DigNum (strict)"() -> ("Value"=w5808:dbl)  [unwired: 2 in, 2 out]
                            n4441 = Divide(x=w5809, y=w5808) -> (x/y=w5810:dbl)
                            n4442 = for {
                              N: w5808 -> [_]
                              tunnel: w5810 -> [w5822]
                              tunnel: w5805 -> [w5819]
                              tunnel: w5802 -> [w5815]
                              i -> [w5817]
                              n4443 = Increment(x=w5817) -> (x+1=w5816:i32)
                              n4444 = Multiply(x=w5822, y=w5816) -> (x*y=w5821:dbl)
                              n4445 = Add(x=w5821, y=w5815) -> (x+y=w5818:dbl)
                              n4446 = property on="Channel" class="Enum (strict)"() -> ("Value"=w5814:T2)  [unwired: 2 in, 2 out]
                              n4447 = Wait (ms)(milliseconds to wait=u32 12) -> ()  [unwired: 1 out]
                              n4448 = call "setLevel.vi"("VISA resource name 2"=w5819, "Source"=Source."Voltage", "Channel"=w5814, "SourceLevel"=w5818) -> ()  [unwired: 1 in, 3 out]
                            }
                          }
                        }
                      }
                      frame #11 {
                        n4449 = Wait (ms)(milliseconds to wait=u32 500) -> ()  [unwired: 1 out]
                      }
                    }
                  }
                  frame "iTC_step" {
                    # "step temperature"
                    n4450 = stacked-sequence {
                      tunnel: w5835 -> [w5842 w5845 w5857]
                      frame #0 {
                        n4451 = property on="iTC_addr_step" class="VISAName"() -> ("Value"=w5844:refnum<visa-resource-name>)  [unwired: 2 in, 2 out]
                        n4452 = Decrement(x=w5842) -> (x-1=w5839:dbl)
                        n4453 = Less Or Equal To 0?(x=w5839) -> (x <= 0?=w5841:bool)
                        n4454 = Select(t=0.0, s=w5841, f=w5839) -> (s? t:f=w5838:dbl)
                        n4455 = call "iTCset.vi"("Set Point"=w5838, "iTCSetCtrl"=iTCsetCtrl."Set VTI Temp", "VISA resource name"=w5844) -> ("VISA resource name out"=w5837:refnum<visa-resource-name>)  [unwired: 5 in, 3 out]
                        n4456 = property on="iTC_addr_step" class="VISAName"("Value"=w5837) -> ()  [unwired: 2 in, 2 out]
                        n4457 = Wait (ms)(milliseconds to wait=u32 200) -> ()  [unwired: 1 out]
                      }
                      frame #1 {
                        n4458 = property on="iTC_addr_step" class="VISAName"() -> ("Value"=w5852:refnum<visa-resource-name>)  [unwired: 2 in, 2 out]
                        n4459 = Less Or Equal To 0?(x=w5845) -> (x <= 0?=w5850:bool)
                        n4460 = Select(t=0.0, s=w5850, f=w5845) -> (s? t:f=w5848:dbl)
                        n4461 = call "iTCset.vi"("Set Point"=w5848, "iTCSetCtrl"=iTCsetCtrl."Set Sample Temp", "VISA resource name"=w5852) -> ("VISA resource name out"=w5847:refnum<visa-resource-name>)  [unwired: 5 in, 3 out]
                        n4462 = property on="iTC_addr_step" class="VISAName"("Value"=w5847) -> ()  [unwired: 2 in, 2 out]
                        n4463 = Wait (ms)(milliseconds to wait=u32 200) -> ()  [unwired: 1 out]
                      }
                      frame #2 {
                        n4464 = Less Or Equal?(x=w5857, y=5.0) -> (x <= y?=w5855:bool)
                        n4465 = Greater Or Equal?(x=w5857, y=3.0) -> (x >= y?=w5854:bool)
                        n4466 = And(x=w5855, y=w5854) -> (x .and. y?=w5853:bool)
                        n4467 = case shown="True" w5853 {
                          tunnel: w5857 -> [w5859 w5869]
                          frame True {
                            n4468 = while {
                              tunnel: w5859 -> [w5861]
                              stop <- w5864 stop-if-true
                              n4469 = property on="iTC_addr_step" class="VISAName"() -> ("Value"=w5868:refnum<visa-resource-name>)  [unwired: 2 in, 2 out]
                              n4470 = Decrement(x=w5861) -> (x-1=w5860:dbl)
                              n4471 = call "iTCread.vi"("VISA resource name"=w5868, "iTCreadCtrl"=iTCreadCtrl."VTI Temp") -> ("number"=w5862:dbl)  [unwired: 5 in, 3 out]
                              n4472 = Subtract(x=w5862, y=w5860) -> (x-y=w5866:dbl)
                              n4473 = property on="Step Channel" class="DigNum (strict)"("Value"=w5862) -> ()  [unwired: 2 in, 2 out]
                              n4474 = property on="Tolerance_Step" class="DigNum (strict)"() -> ("Value"=w5863:dbl)  [unwired: 2 in, 2 out]
                              n4475 = Absolute Value(x=w5866) -> (abs(x)=w5865:dbl)
                              n4476 = Less?(x=w5865, y=w5863) -> (x < y?=w5864:bool)
                              n4477 = property on="at field" class="Bool (strict)"("Value"=w5864) -> ()  [unwired: 2 in, 2 out]
                            }
                          }
                          frame False {
                            n4478 = while {
                              tunnel: w5869 -> [w5875]
                              stop <- w5872 stop-if-true
                              n4479 = property on="iTC_addr_step" class="VISAName"() -> ("Value"=w5877:refnum<visa-resource-name>)  [unwired: 2 in, 2 out]
                              n4480 = call "iTCread.vi"("VISA resource name"=w5877, "iTCreadCtrl"=iTCreadCtrl."Sample Temp") -> ("number"=w5870:dbl)  [unwired: 5 in, 3 out]
                              n4481 = property on="Tolerance_Step" class="DigNum (strict)"() -> ("Value"=w5871:dbl)  [unwired: 2 in, 2 out]
                              n4482 = Subtract(x=w5870, y=w5875) -> (x-y=w5874:dbl)
                              n4483 = property on="Step Channel" class="DigNum (strict)"("Value"=w5870) -> ()  [unwired: 2 in, 2 out]
                              n4484 = Absolute Value(x=w5874) -> (abs(x)=w5873:dbl)
                              n4485 = Less?(x=w5873, y=w5871) -> (x < y?=w5872:bool)
                              n4486 = property on="at field" class="Bool (strict)"("Value"=w5872) -> ()  [unwired: 2 in, 2 out]
                            }
                          }
                        }
                      }
                    }
                  }
                  frame "2461_Curr" {
                    n4487 = property on="2461_addr_step" class="VISAName"() -> ("Value"=w5878:refnum<visa-resource-name>)  [unwired: 2 in, 2 out]
                    n4488 = property on="Step Channel" class="DigNum (strict)"() -> ("Value"=w5881:dbl)  [unwired: 2 in, 2 out]
                    n4489 = property on="Mini steps" class="DigNum (strict)"() -> ("Value"=w5880:dbl)  [unwired: 2 in, 2 out]
                    n4490 = Subtract(x=w5879, y=w5881) -> (x-y=w5882:dbl)
                    n4491 = Divide(x=w5882, y=w5880) -> (x/y=w5883:dbl)
                    n4492 = for {
                      N: w5880 -> [_]
                      tunnel: w5881 -> [w5892]
                      tunnel: w5883 -> [w5891]
                      tunnel: w5878 -> [w5886]
                      i -> [w5888]
                      w5885 = u16 1 items=["Volts", "Current"] ("Function (0: Volts)")
                      n4493 = Increment(x=w5888) -> (x+1=w5887:i32)
                      n4494 = Multiply(x=w5891, y=w5887) -> (x*y=w5890:dbl)
                      n4495 = Add(x=w5890, y=w5892) -> (x+y=w5884:dbl)
                      n4496 = call <instrlib>:"Configure Source Level.vi"("Source Level (1.0)"=w5884, "Function (0: Volts)"=w5885, "VISA resource name"=w5886) -> ()  [unwired: 7 in, 2 out]
                      n4497 = Wait (ms)(milliseconds to wait=u32 12) -> ()  [unwired: 1 out]
                      n4498 = property on="Current Step Value" class="DigNum (strict)"("Value"=w5884) -> ()  [unwired: 2 in, 2 out]
                    }
                  }
                }
              }
              frame #1 {
                n4499 = property on="Current Step Value" class="DigNum (strict)"() -> ("Value"=w5897:dbl)  [unwired: 2 in, 2 out]
                n4500 = property on="Change Sweep Range" class="Bool (strict)"() -> ("Value"=w5893:bool)  [unwired: 2 in, 2 out]
                n4501 = property on="Step Channel" class="DigNum (strict)"("Value"=w5897) -> ()  [unwired: 2 in, 2 out]
                n4502 = case shown="True" w5893 {
                  frame False {
                  }
                  frame True {
                    n4503 = property on="Table Index" class="DigNum (strict)"() -> ("Value"=w5898:dbl)  [unwired: 2 in, 2 out]
                    n4504 = property on="Down          Up" class="Tbl (strict)"() -> ("Value"=w5904:string[][])  [unwired: 2 in, 2 out]
                    n4505 = Index Array(array=w5904, index (row)=w5898, index (col)=0 ("disabled index (col)")) -> (element=w5902:string)
                    n4506 = Index Array(array=w5904, index (row)=w5898, index (col)=1 ("disabled index (col)")) -> (element=w5899:string)
                    n4507 = Fract/Exp String To Number(string=w5902) -> (number=w5901:dbl)  [unwired: 3 in, 1 out]
                    n4508 = Fract/Exp String To Number(string=w5899) -> (number=w5900:dbl)  [unwired: 3 in, 1 out]
                    n4509 = property on="lower limit" class="DigNum (strict)"("Value"=w5901) -> ()  [unwired: 2 in, 2 out]
                    n4510 = property on="upper limit" class="DigNum (strict)"("Value"=w5900) -> ()  [unwired: 2 in, 2 out]
                  }
                }
                n4511 = property on="Wait Between Step(s)" class="DigNum (strict)"() -> ("Value"=w5896:i32)  [unwired: 2 in, 2 out]
                n4512 = Multiply(x=w5896, y=1000) -> (x*y=w5894:i32)
                n4513 = Wait (ms)(milliseconds to wait=w5894) -> ()  [unwired: 1 out]
              }
              frame #2 {
                n4514 = property on="Sweep Direction" class="Str"() -> ("Value"=w5906:string)  [unwired: 2 in, 2 out]
                n4515 = case shown="\"Ramp Down\", Default" w5906 {
                  frame "Sweep Down" {
                    n4516 = property on="Up Rate" class="DigNum (strict)" props=["Value"]() -> ()  [unwired: 2 in, 3 out]
                    n4517 = property on="upper limit" class="DigNum (strict)" props=["Value"]() -> ()  [unwired: 2 in, 3 out]
                    n4518 = property on="Down Rate" class="DigNum (strict)"() -> ("Value"=w5907:dbl)  [unwired: 2 in, 2 out]
                    n4519 = property on="lower limit" class="DigNum (strict)"() -> ("Value"=w5908:dbl)  [unwired: 2 in, 2 out]
                    n4520 = property on="sweep to:" class="DigNum (strict)"("Value"=w5908) -> ()  [unwired: 2 in, 2 out]
                    n4521 = property on="sweep rate, /min" class="DigNum (strict)"("Value"=w5907) -> ()  [unwired: 2 in, 2 out]
                  }
                  frame "Ramp Down", Default {
